vi "sv_Octave Range to Band Number.vi"(1 "frequency range":T1={"low band"=enum."1000 Hz", "high band"=enum."1000 Hz"}) -> (0 "band number":cluster{"low band":i32, "high band":i32})   [LabVIEW 2017, in "SoundVib_Octave_2014 standard.lvlib"]
doc: "Converts the selected octave frequency range to the corresponding band number.\nThe band number is based on the low and high bands specified in the frequency range cluster. A value of 0 corresponds to the reference frequency of the audio-frequency range, 1 kHz. Each successive value corresponds to the next octave band. Positive values cover the range above 1 kHz, and negative values cover the range below 1 kHz.\nThe frequency range cluster uses a pre-defined list of frequencies from 16 Hz to 16 kHz, in octave steps. If you need to use any other specific frequency outside of this frequency range, use the Frequency Range to Band Number VI instead."
uses:
  <vilib>/addons/Sound and Vibration/svt_Octave/SoundVib_Octave_2014 standard.lvlib
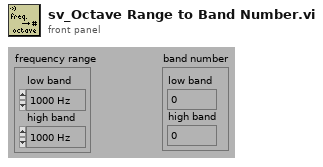
[diagram p1: front panel]
types:
  T1 = cluster{"low band":enum16{"16 Hz", "31.5 Hz", "63 Hz", "125 Hz", "250 Hz", "500 Hz", "1000 Hz", "2000 Hz", "4000 Hz", "8000 Hz", "16000 Hz"}, "high band":enum16{"16 Hz", "31.5 Hz", "63 Hz", "125 Hz", "250 Hz", "500 Hz", "1000 Hz", "2000 Hz", "4000 Hz", "8000 Hz", "16000 Hz"}}
  T2 = enum16{"16 Hz", "31.5 Hz", "63 Hz", "125 Hz", "250 Hz", "500 Hz", "1000 Hz", "2000 Hz", "4000 Hz", "8000 Hz", "16000 Hz"}
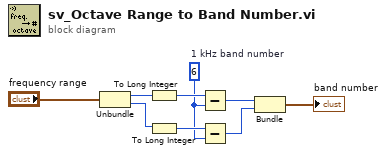
[diagram p0: block diagram]
diagram:
  w4 = 6  # 1 kHz band number
  n1 = Unbundle("frequency range") -> ("low band"=w8:T2, "high band"=w9:T2)
  n2 = To Long Integer(number=w8) -> (32bit integer=w6:i32)
  n3 = To Long Integer(number=w9) -> (32bit integer=w7:i32)
  n4 = Subtract(x=w6, y=w4) -> (x-y=w3:i32)
  n5 = Subtract(x=w7, y=w4) -> (x-y=w2:i32)
  n6 = Bundle(w3, w2) -> (→"band number":cluster{i32, i32})  [unwired: 1 in]
